vi "plant_structure.vi"(9 "Dataflow":errorcluster, 10 "Pause":refnum<vi>, 11 "Stop":refnum<vi>) -> ()   [LabVIEW 2019]
uses:
  lib/libSimulationControl/libSimulationControl.lvlib
panel:
  out "Dataflow Out":errorcluster
  # "*******************************************************************\nBiogas Plant Control\n\nAuthor: Paul Zügel\nGCSC-Frankfurt am Main 2020\n\n*******************************************************************"
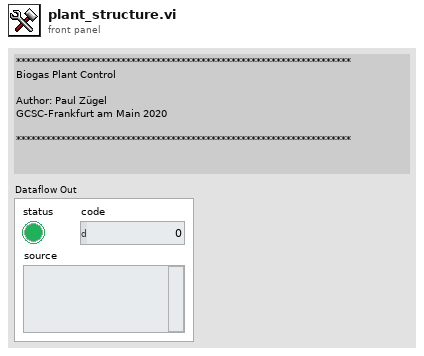
[diagram p1: front panel]
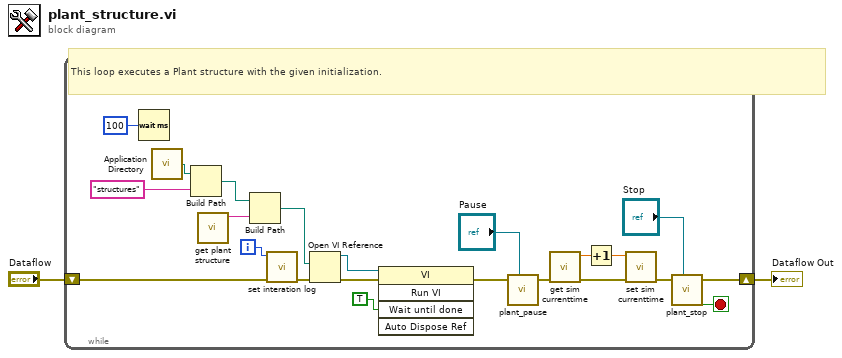
[diagram p0: block diagram]
diagram:
  n1 = while {
    shift-right: [w21] -> w1
    shift-left: "Dataflow" -> [w3]
    i -> [w20]
    stop <- w11 stop-if-true
    # "This loop executes a Plant structure with the given initialization."
    n2 = Wait (ms)(milliseconds to wait=u32 100) -> ()  [unwired: 1 out]
    n3 = call <vilib>:"Application Directory.vi"() -> ("Application Directory"=w4:path)
    n4 = Build Path(base path=w4, name or relative path="structures") -> (appended path=w17:path)
    n5 = call "get plant structure.vi"() -> ("function return"=w19:string)  [unwired: 10 in, 1 out]
    n6 = Build Path(base path=w17, name or relative path=w19) -> (appended path=w16:path)
    n7 = call "set interation log.vi"("error in (no error)"=w3, "iter"=w20) -> ("error out"=w6:errorcluster)  [unwired: 9 in]
    n8 = Open VI Reference(vi path=w16, error in (no error)=w6) -> (vi reference=w12:refnum<vi>, error out=w15:errorcluster)  [unwired: 4 in]
    n9 = invoke class="VI" method="Run VI"(reference=w12, error in=w15, "Wait until done"=TRUE ("Wait Until Done")) -> (error out=w14:errorcluster)  [unwired: 2 in, 4 out]
    n10 = call "plant_pause.vi"("Dataflow In"=w14, "Pause"="Pause") -> ("Dataflow Out"=w8:errorcluster)  [unwired: 5 in]
    n11 = call "get sim currenttime.vi"("error in (no error)"=w8) -> ("error out"=w10:errorcluster, "current_time"=w5:dbl)  [unwired: 9 in]
    n12 = Increment(x=w5) -> (x+1=w9:dbl)
    n13 = call "set sim currenttime.vi"("error in (no error)"=w10, "time"=w9) -> ("error out"=w7:errorcluster)  [unwired: 9 in]
    n14 = call "plant_stop.vi"("Dataflow In"=w7, "Stop In"="Stop") -> ("Stop Out"=w11:bool, "Dataflow Out"=w21:errorcluster)  [unwired: 4 in]
  }
  "Dataflow Out" <- w1
